vi "Replot.vi"(8 "error in (no error)":errorcluster, 11 "MagLabGraph in":refnum<class "MagLabGraph.lvclass">) -> (0 "error out":errorcluster, 3 "MagLabGraph out":refnum<class "MagLabGraph.lvclass">)   [LabVIEW 2015, in "MagLabGraph.lvclass"]
uses:
  MagLabGraph.lvclass
  MagLabGraph.lvclass/MagLabGraph.ctl
  Mag Lab Error Handler/Mag Lab Error Handler.lvclass
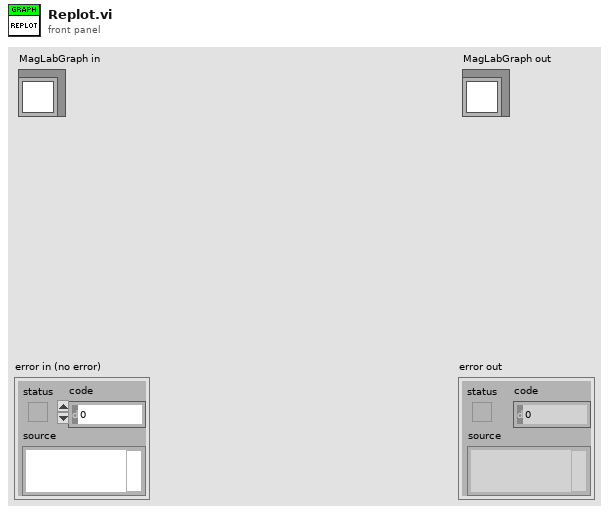
[diagram p1: front panel]
types:
  T1 = typedef "Data reduction.ctl" = cluster{"Clip time":bool, "Tiime 0":dbl, "Time 1":dbl, "Maximum data points":i32, "Decimation method":enum16{"coerce", "linear", "spline", "Min-Max", "Average"}}
  T2 = cluster{"File Path Control":path, "Group":string, "Channel":string, "Abbreviated":string}[]
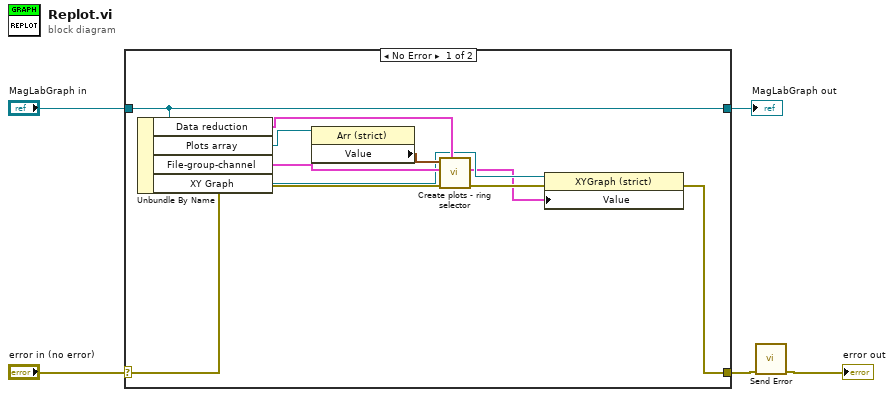
[diagram p0: block diagram]
diagram:
  n1 = case shown="No Error" "error in (no error)" {
    selector: "error in (no error)" -> [w10 w17]
    tunnel: [w8 w17] -> w2
    tunnel: [w15 w16] -> w3
    tunnel: "MagLabGraph in" -> [w15 w16]
    frame No Error {
      n2 = Unbundle By Name(w15) -> ("Data reduction"=w11:T1, "Plots array"=w14:refnum<vi>, "File-group-channel"=w12:T2, "XY Graph"=w7:refnum<vi>)
      n3 = property class="Arr (strict)"(reference=w14) -> ("Value"=w13:cluster{"X":u16, "Y":u16}[])  [unwired: 1 in, 2 out]
      n4 = call "Create plots - ring selector.vi"("Data reduction"=w11, "Error In"=w10, "File-group-channel"=w12, "Plots  selector"=w13) -> ("Error Out"=w9:errorcluster, "Plots"=w6:cluster{dbl[], dbl[]}[])  [unwired: 6 in]
      n5 = property class="XYGraph (strict)"(reference=w7, error in=w9, "Value"=w6) -> (error out=w8:errorcluster)  [unwired: 1 out]
    }
    frame Error {
    }
  }
  "MagLabGraph out" <- w3
  n6 = call "Send Error.vi"("error in (no error)"=w2) -> ("error out"=→"error out":errorcluster)  [unwired: 9 in, 1 out]
